vi "CTRE_PigeonIMU_Global.vi"(4 "32-bit Frame":i32, 6 "Set Boolean":bool, 7 "Write After Receive":T2={"PigeonState"=enum."NoComm", "FusedHeading"={"Heading"=0.0, "Valid?"=TRUE, "Fusing?"=TRUE}, "YPR"={"Yaw"=0.0, "Pitch"=0.0, "Roll"=0.0}, "Compass"={"Heading"=0.0, "Magnitude"=0.0, "Absolute Heading"=0.0}, "Accelerometer"={"Biased"={"X"=0, "Y"=0, "Z"=0, "Norm"=0}, "Angles"={"XZ Tilt"=0.0, "YZ Tilt"=0.0, "XY Tilt"=0.0}}, "Magnetometer"={"Raw"={"X"=0, "Y"=0, "Z"=0}, "Biased"={"X"=0, "Y"=0, "Z"=0}}, "Gyro"={"X"=0.0, "Y"=0.0, "Z"=0.0, "Norm"=0.0}, "6D Quaternian"={"W"=0.0, "X"=0.0, "Y"=0.0, "Z"=0.0}, "Temp. (C)"=0.0, "UpTime"=0, "StartupStatus"={"ResetCount"=0, "ResetFlags"=0, "FirmwareVersion"=0, "HasReset?"=TRUE}, "Calibration"={"CurrentMode"=0, "LastCalError"=0, "CalBooting?"=TRUE}, "CAN Error"={"status"=FALSE, "code"=0, "source"=""}, "AccumGyro"={"X"=0.0, "Y"=0.0, "Z"=0.0}, "Usage Frame"=0} {"Calibration"."CurrentMode" items=["BootTareGryoAccel"=0, "Temperature"=1, "Magnetometer12Pt"=2, "Magnetometer360"=3, "Accelerometer"=5]}, 8 "Set Number":dbl, 10 "Operation":T1, 11 "Device ID (0)":u8) -> (1 "Get All":T2={"PigeonState"=enum."NoComm", "FusedHeading"={"Heading"=0.0, "Valid?"=TRUE, "Fusing?"=TRUE}, "YPR"={"Yaw"=0.0, "Pitch"=0.0, "Roll"=0.0}, "Compass"={"Heading"=0.0, "Magnitude"=0.0, "Absolute Heading"=0.0}, "Accelerometer"={"Biased"={"X"=0, "Y"=0, "Z"=0, "Norm"=0}, "Angles"={"XZ Tilt"=0.0, "YZ Tilt"=0.0, "XY Tilt"=0.0}}, "Magnetometer"={"Raw"={"X"=0, "Y"=0, "Z"=0}, "Biased"={"X"=0, "Y"=0, "Z"=0}}, "Gyro"={"X"=0.0, "Y"=0.0, "Z"=0.0, "Norm"=0.0}, "6D Quaternian"={"W"=0.0, "X"=0.0, "Y"=0.0, "Z"=0.0}, "Temp. (C)"=0.0, "UpTime"=0, "StartupStatus"={"ResetCount"=0, "ResetFlags"=0, "FirmwareVersion"=0, "HasReset?"=TRUE}, "Calibration"={"CurrentMode"=0, "LastCalError"=0, "CalBooting?"=TRUE}, "CAN Error"={"status"=FALSE, "code"=0, "source"=""}, "AccumGyro"={"X"=0.0, "Y"=0.0, "Z"=0.0}, "Usage Frame"=0} {"Calibration"."CurrentMode" items=["BootTareGryoAccel"=0, "Temperature"=1, "Magnetometer12Pt"=2, "Magnetometer360"=3, "Accelerometer"=5]}, 3 "Device ID Out":u8, 5 "Read For Send":T5)   [LabVIEW 2016]
uses:
  <vilib>/Rock Robotics/WPI/ThirdParty/Sensors/Pigeon IMU/CTRE_PigeonIMU_GlobalControl.ctl
  <vilib>/Rock Robotics/WPI/ThirdParty/Sensors/Pigeon IMU/CTRE_PigeonIMU_GlobalStatus.ctl
  <vilib>/Rock Robotics/WPI/ThirdParty/Sensors/Pigeon IMU/CTRE_PigeonIMU_PigeonState.ctl
  <vilib>/Rock Robotics/WPI/ThirdParty/Sensors/Pigeon IMU/CTRE_PigeonIMU_CalibrationMode.ctl
  <vilib>/Rock Robotics/WPI/ThirdParty/Sensors/Pigeon IMU/CTRE_PigeonIMU_GlobalOps.ctl
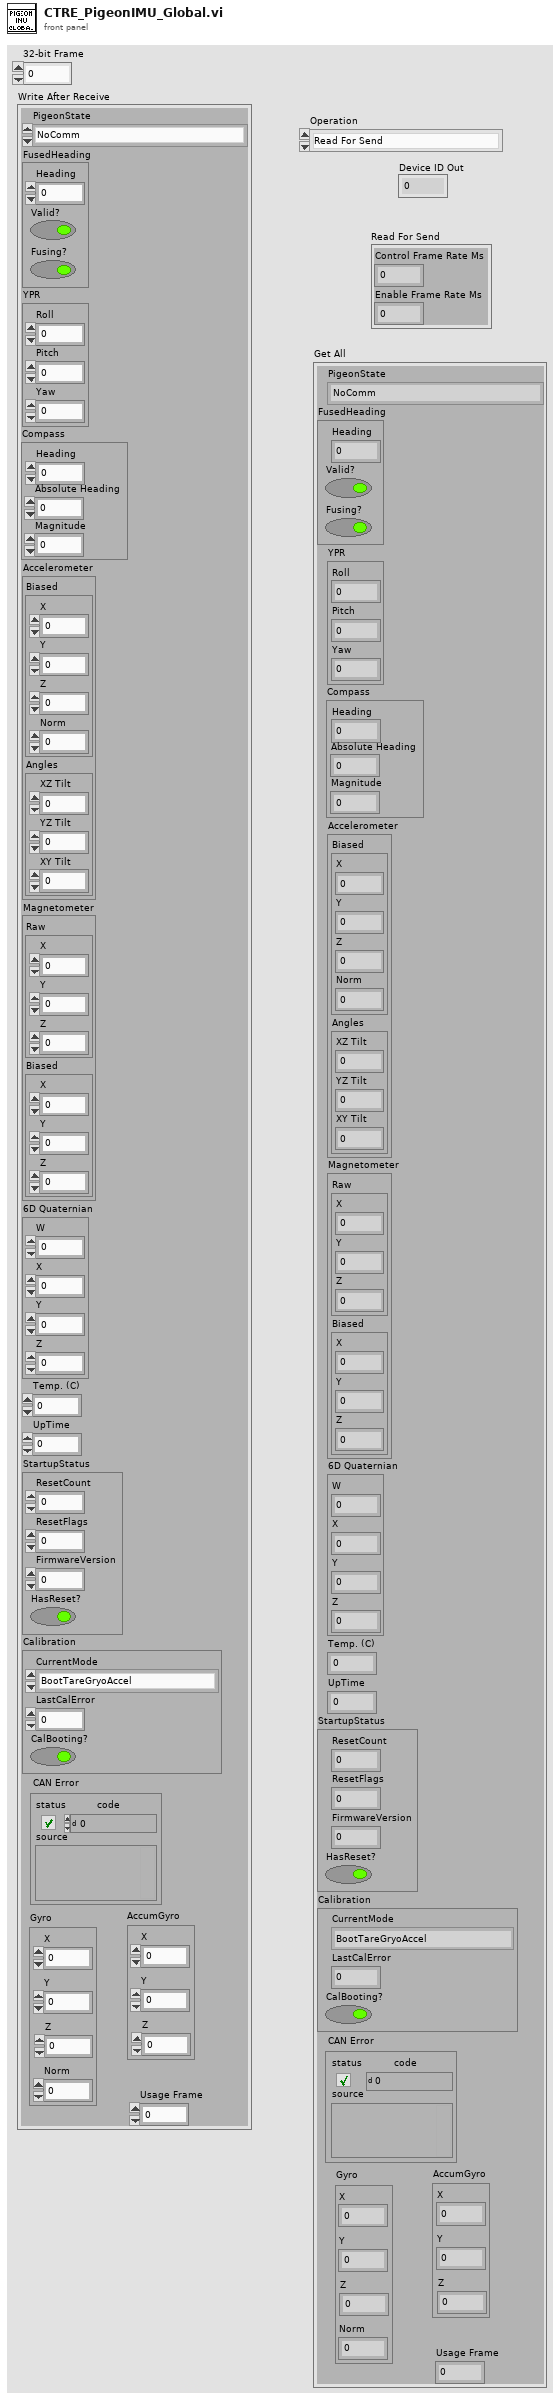
[diagram p1: front panel]
types:
  T1 = typedef "CTRE_PigeonIMU_GlobalOps.ctl" = enum16{"Read For Send", "Write Error", "Get All", "Set Control Frame Rate", "Set Enable Frame Rate", "Write After Receive Fused Heading", "Write After Receive YPR", "Write After Receive Status", "Write After Receive Raw Magnetomoter", "Write After Receive Biased Magnetometer", "Write After Receive Biased Accelerometer", "Write After Receive Gyro", "Write After Receive Acceleromter Angles", "Write After Receive Startup Status", "Write After Receive Compass", "Write After Receive Quaternian", "Write After Receive AccumGyro", "Set Usage Frame"}
  T2 = typedef "CTRE_PigeonIMU_GlobalStatus.ctl" = cluster{"PigeonState":T3, "FusedHeading":cluster{"Heading":dbl, "Valid?":bool, "Fusing?":bool}, "YPR":cluster{"Yaw":dbl, "Pitch":dbl, "Roll":dbl}, "Compass":cluster{"Heading":dbl, "Magnitude":dbl, "Absolute Heading":dbl}, "Accelerometer":cluster{"Biased":cluster{"X":i16, "Y":i16, "Z":i16, "Norm":i16}, "Angles":cluster{"XZ Tilt":dbl, "YZ Tilt":dbl, "XY Tilt":dbl}}, "Magnetometer":cluster{"Raw":cluster{"X":i16, "Y":i16, "Z":i16}, "Biased":cluster{"X":i16, "Y":i16, "Z":i16}}, "Gyro":cluster{"X":dbl, "Y":dbl, "Z":dbl, "Norm":dbl}, "6D Quaternian":cluster{"W":dbl, "X":dbl, "Y":dbl, "Z":dbl}, "Temp. (C)":dbl, "UpTime":u32, "StartupStatus":cluster{"ResetCount":i32, "ResetFlags":i32, "FirmwareVersion":i32, "HasReset?":bool}, "Calibration":cluster{"CurrentMode":T4, "LastCalError":i32, "CalBooting?":bool}, "CAN Error":errorcluster, "AccumGyro":cluster{"X":dbl, "Y":dbl, "Z":dbl}, "Usage Frame":u32}
  T3 = typedef "CTRE_PigeonIMU_PigeonState.ctl" = enum16{"NoComm", "Initializing", "Ready", "UserCalibration"}
  T4 = typedef "CTRE_PigeonIMU_CalibrationMode.ctl" = u16
  T5 = typedef "CTRE_PigeonIMU_GlobalControl.ctl" = cluster{"Control Frame Rate Ms":i32, "Enable Frame Rate Ms":i32}
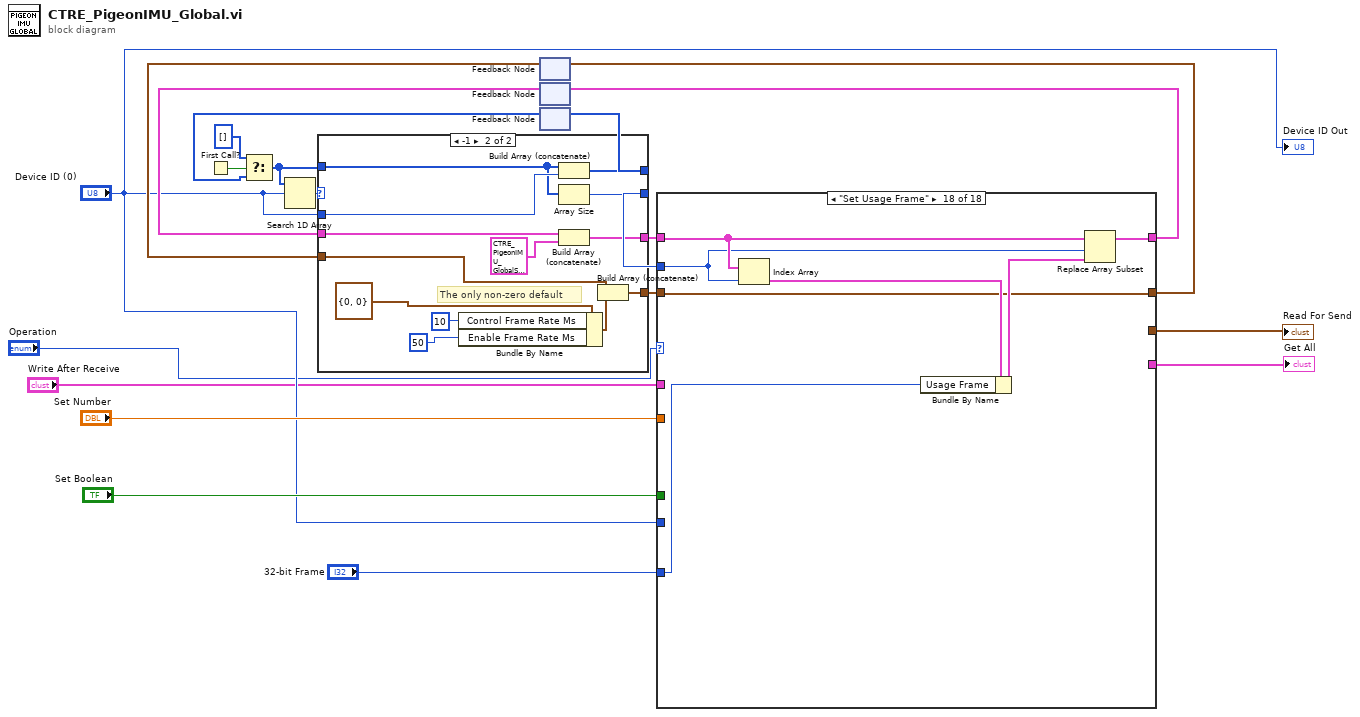
[diagram p0: block diagram]
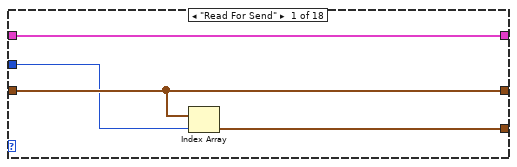
[diagram p2: hidden frame]
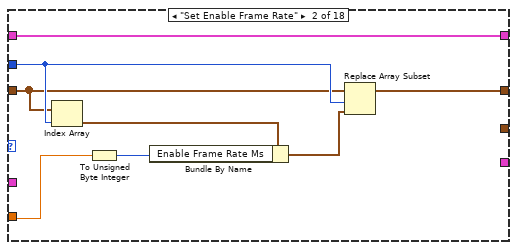
[diagram p3: hidden frame]
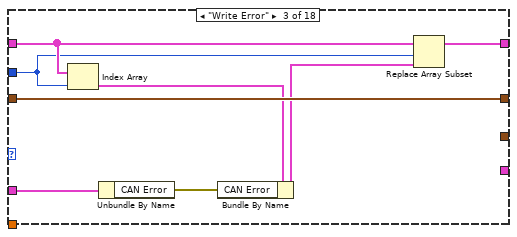
[diagram p4: hidden frame]
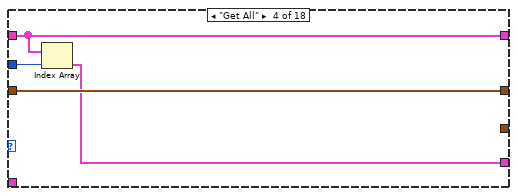
[diagram p5: hidden frame]
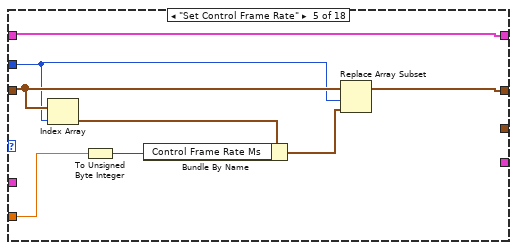
[diagram p6: hidden frame]
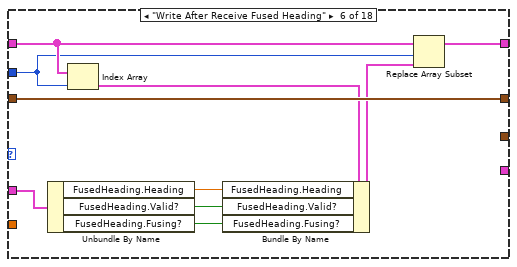
[diagram p7: hidden frame]
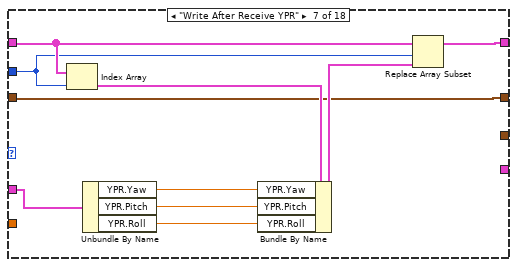
[diagram p8: hidden frame]
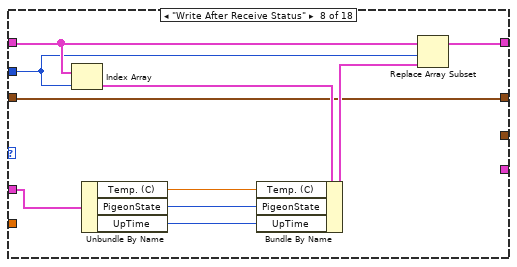
[diagram p9: hidden frame]
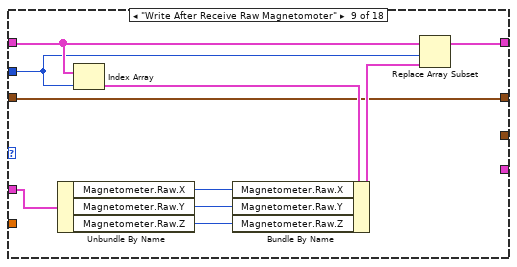
[diagram p10: hidden frame]
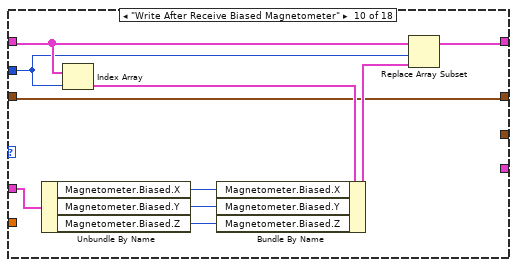
[diagram p11: hidden frame]
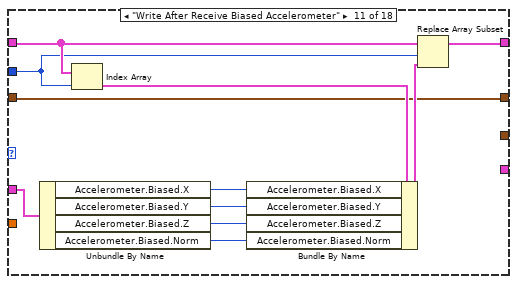
[diagram p12: hidden frame]
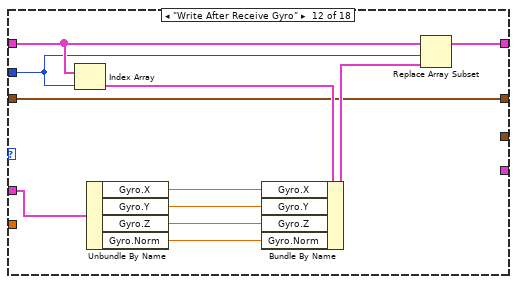
[diagram p13: hidden frame]
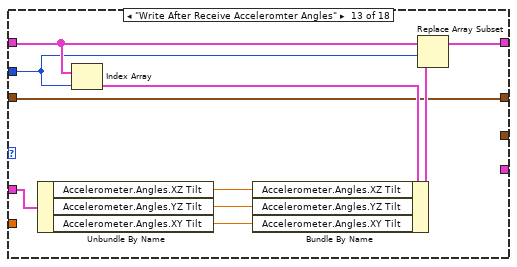
[diagram p14: hidden frame]
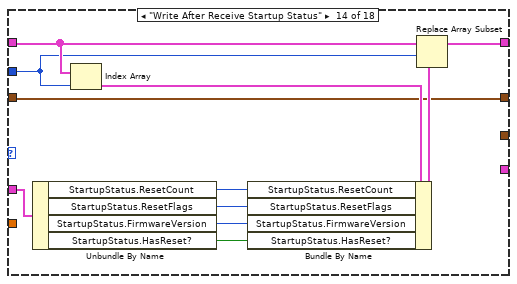
[diagram p15: hidden frame]
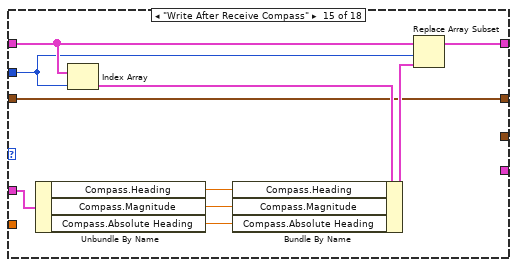
[diagram p16: hidden frame]
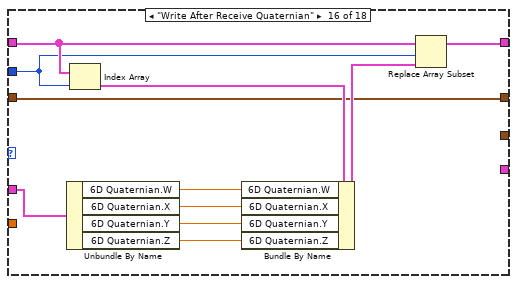
[diagram p17: hidden frame]
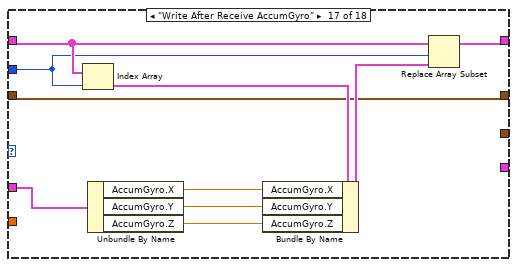
[diagram p18: hidden frame]
diagram:
  n1 = First Call?() -> (First Call?: T/F=w21:bool)
  n2 = feedback #1() -> (w14:T5[])  [unwired: 1 in]
  n3 = feedback #2() -> (w15:T2[])  [unwired: 1 in]
  n4 = feedback #3() -> (w19:u8[])  [unwired: 1 in]
  n5 = Select(t=u8[] [], s=w21, f=w19) -> (s? t:f=w17:u8[])
  n6 = Search 1D Array(1D array=w17, element="Device ID (0)") -> (index of element=w16:i32)  [unwired: 1 in]
  n7 = case shown="-1" w16 {
    selector: w16 -> [w22 _]
    tunnel: [w25 w38] -> w18
    tunnel: "Device ID (0)" -> [_ w37]
    tunnel: w17 -> [w25 w32]
    tunnel: w15 -> [w24 w36]
    tunnel: w14 -> [w23 w35]
    tunnel: [w24 w34] -> w12
    tunnel: [w23 w33] -> w10
    tunnel: [w22 w31] -> w9
    frame Default {
    }
    frame -1 {
      # "The only non-zero default"
      n8 = Bundle By Name(cluster=T5 {"Control Frame Rate Ms"=0, "Enable Frame Rate Ms"=0} ("PigeonIMU Control"), "Control Frame Rate Ms"=u8 10, "Enable Frame Rate Ms"=u8 50) -> (w30:T5)
      n9 = Build Array (concatenate)(w32, w37) -> (w38:u8[])
      n10 = Array Size(array=w32) -> (size(s)=w31:i32)
      n11 = Build Array (concatenate)(w36, T2 {"PigeonState"=enum."NoComm", "FusedHeading"={"Heading"=0.0, "Valid?"=TRUE, "Fusing?"=TRUE}, "YPR"={"Yaw"=0.0, "Pitch"=0.0, "Roll"=0.0}, "Compass"={"Heading"=0.0, "Magnitude"=0.0, "Absolute Heading"=0.0}, "Accelerometer"={"Biased"={"X"=0, "Y"=0, "Z"=0, "Norm"=0}, "Angles"={"XZ Tilt"=0.0, "YZ Tilt"=0.0, "XY Tilt"=0.0}}, "Magnetometer"={"Raw"={"X"=0, "Y"=0, "Z"=0}, "Biased"={"X"=0, "Y"=0, "Z"=0}}, "Gyro"={"X"=0.0, "Y"=0.0, "Z"=0.0, "Norm"=0.0}, "6D Quaternian"={"W"=0.0, "X"=0.0, "Y"=0.0, "Z"=0.0}, "Temp. (C)"=0.0, "UpTime"=0, "StartupStatus"={"ResetCount"=0, "ResetFlags"=0, "FirmwareVersion"=0, "HasReset?"=TRUE}, "Calibration"={"CurrentMode"=0, "LastCalError"=0, "CalBooting?"=TRUE}, "CAN Error"={"status"=FALSE, "code"=0, "source"=""}, "AccumGyro"={"X"=0.0, "Y"=0.0, "Z"=0.0}, "Usage Frame"=0} ("PigeonIMU Status")) -> (w34:T2[])
      n12 = Build Array (concatenate)(w35, w30) -> (w33:T5[])
    }
  }
  n13 = feedback-in #3(w18) -> ()
  n14 = case shown="\"Set Usage Frame\"" "Operation" {
    tunnel: [w42 w44 w57 w60 w66 w79 w84 w94 w104 w114 w125 w136 w146 w157 w168 w179 w188 w197] -> w13
    tunnel: w12 -> [w42 w44 w56 w60 w66 w78 w85 w95 w105 w115 w126 w137 w147 w158 w170 w181 w189 w199]
    tunnel: [w41 w43 w58 w62 w68 w80 w83 w92 w102 w112 w123 w134 w145 w155 w167 w178 w186 w196] -> w11
    tunnel: w10 -> [w41 w45 w58 w62 w69 w80 w83 w92 w102 w112 w123 w134 w145 w155 w167 w178 w186 w196]
    tunnel: w9 -> [w40 w46 w55 w61 w67 w77 w82 w93 w103 w113 w124 w135 w143 w156 w169 w180 w187 w198]
    tunnel: [w39 _ _ _ _ _ _ _ _ _ _ _ _ _ _ _ _ _] -> w5
    tunnel: "Write After Receive" -> [_ _ w52 _ _ w74 w81 w91 w101 w111 w122 w133 w144 w154 w166 w177 w185 _]
    tunnel: "Set Number" -> [_ w47 _ _ w64 _ _ _ _ _ _ _ _ _ _ _ _ _]
    tunnel: [_ _ _ w59 _ _ _ _ _ _ _ _ _ _ _ _ _ _] -> w4
    tunnel: "Set Boolean" -> [_ _ _ _ _ _ _ _ _ _ _ _ _ _ _ _ _ _]
    tunnel: "Device ID (0)" -> [_ _ _ _ _ _ _ _ _ _ _ _ _ _ _ _ _ _]
    tunnel: "32-bit Frame" -> [_ _ _ _ _ _ _ _ _ _ _ _ _ _ _ _ _ w195]
    frame "Read For Send" {
      n15 = Index Array(array=w41, index=w40) -> (element=w39:T5)
    }
    frame "Set Enable Frame Rate" {
      n16 = Index Array(array=w45, index=w46) -> (element=w49:T5)
      n17 = To Unsigned Byte Integer(number=w47) -> (unsigned 8bit integer=w48:u8)
      n18 = Bundle By Name(cluster=w49, "Enable Frame Rate Ms"=w48) -> (w50:T5)
      n19 = Replace Array Subset(array=w45, new element=w50, index=w46) -> (w43:T5[])
    }
    frame "Write Error" {
      n20 = Index Array(array=w56, index=w55) -> (element=w54:T2)
      n21 = Unbundle By Name(w52) -> ("CAN Error"=w51:errorcluster)
      n22 = Bundle By Name(cluster=w54, "CAN Error"=w51) -> (w53:T2)
      n23 = Replace Array Subset(array=w56, new element=w53, index=w55) -> (w57:T2[])
    }
    frame "Get All" {
      n24 = Index Array(array=w60, index=w61) -> (element=w59:T2)
    }
    frame "Set Control Frame Rate" {
      n25 = Index Array(array=w69, index=w67) -> (element=w65:T5)
      n26 = To Unsigned Byte Integer(number=w64) -> (unsigned 8bit integer=w63:u8)
      n27 = Bundle By Name(cluster=w65, "Control Frame Rate Ms"=w63) -> (w70:T5)
      n28 = Replace Array Subset(array=w69, new element=w70, index=w67) -> (w68:T5[])
    }
    frame "Write After Receive Fused Heading" {
      n29 = Unbundle By Name(w74) -> ("FusedHeading.Heading"=w73:dbl, "FusedHeading.Valid?"=w72:bool, "FusedHeading.Fusing?"=w71:bool)
      n30 = Index Array(array=w78, index=w77) -> (element=w76:T2)
      n31 = Bundle By Name(cluster=w76, "FusedHeading.Heading"=w73, "FusedHeading.Valid?"=w72, "FusedHeading.Fusing?"=w71) -> (w75:T2)
      n32 = Replace Array Subset(array=w78, new element=w75, index=w77) -> (w79:T2[])
    }
    frame "Write After Receive YPR" {
      n33 = Index Array(array=w85, index=w82) -> (element=w86:T2)
      n34 = Unbundle By Name(w81) -> ("YPR.Yaw"=w88:dbl, "YPR.Pitch"=w89:dbl, "YPR.Roll"=w90:dbl)
      n35 = Bundle By Name(cluster=w86, "YPR.Yaw"=w88, "YPR.Pitch"=w89, "YPR.Roll"=w90) -> (w87:T2)
      n36 = Replace Array Subset(array=w85, new element=w87, index=w82) -> (w84:T2[])
    }
    frame "Write After Receive Status" {
      n37 = Index Array(array=w95, index=w93) -> (element=w100:T2)
      n38 = Unbundle By Name(w91) -> ("Temp. (C)"=w98:dbl, "PigeonState"=w97:T3, "UpTime"=w96:u32)
      n39 = Bundle By Name(cluster=w100, "Temp. (C)"=w98, "PigeonState"=w97, "UpTime"=w96) -> (w99:T2)
      n40 = Replace Array Subset(array=w95, new element=w99, index=w93) -> (w94:T2[])
    }
    frame "Write After Receive Raw Magnetomoter" {
      n41 = Unbundle By Name(w101) -> ("Magnetometer.Raw.X"=w108:i16, "Magnetometer.Raw.Y"=w107:i16, "Magnetometer.Raw.Z"=w106:i16)
      n42 = Index Array(array=w105, index=w103) -> (element=w110:T2)
      n43 = Bundle By Name(cluster=w110, "Magnetometer.Raw.X"=w108, "Magnetometer.Raw.Y"=w107, "Magnetometer.Raw.Z"=w106) -> (w109:T2)
      n44 = Replace Array Subset(array=w105, new element=w109, index=w103) -> (w104:T2[])
    }
    frame "Write After Receive Biased Magnetometer" {
      n45 = Unbundle By Name(w111) -> ("Magnetometer.Biased.X"=w118:i16, "Magnetometer.Biased.Y"=w117:i16, "Magnetometer.Biased.Z"=w116:i16)
      n46 = Index Array(array=w115, index=w113) -> (element=w120:T2)
      n47 = Bundle By Name(cluster=w120, "Magnetometer.Biased.X"=w118, "Magnetometer.Biased.Y"=w117, "Magnetometer.Biased.Z"=w116) -> (w119:T2)
      n48 = Replace Array Subset(array=w115, new element=w119, index=w113) -> (w114:T2[])
    }
    frame "Write After Receive Biased Accelerometer" {
      n49 = Unbundle By Name(w122) -> ("Accelerometer.Biased.X"=w129:i16, "Accelerometer.Biased.Y"=w128:i16, "Accelerometer.Biased.Z"=w127:i16, "Accelerometer.Biased.Norm"=w121:i16)
      n50 = Index Array(array=w126, index=w124) -> (element=w131:T2)
      n51 = Bundle By Name(cluster=w131, "Accelerometer.Biased.X"=w129, "Accelerometer.Biased.Y"=w128, "Accelerometer.Biased.Z"=w127, "Accelerometer.Biased.Norm"=w121) -> (w130:T2)
      n52 = Replace Array Subset(array=w126, new element=w130, index=w124) -> (w125:T2[])
    }
    frame "Write After Receive Gyro" {
      n53 = Index Array(array=w137, index=w135) -> (element=w142:T2)
      n54 = Unbundle By Name(w133) -> ("Gyro.X"=w140:dbl, "Gyro.Y"=w139:dbl, "Gyro.Z"=w138:dbl, "Gyro.Norm"=w132:dbl)
      n55 = Bundle By Name(cluster=w142, "Gyro.X"=w140, "Gyro.Y"=w139, "Gyro.Z"=w138, "Gyro.Norm"=w132) -> (w141:T2)
      n56 = Replace Array Subset(array=w137, new element=w141, index=w135) -> (w136:T2[])
    }
    frame "Write After Receive Acceleromter Angles" {
      n57 = Unbundle By Name(w144) -> ("Accelerometer.Angles.XZ Tilt"=w150:dbl, "Accelerometer.Angles.YZ Tilt"=w151:dbl, "Accelerometer.Angles.XY Tilt"=w152:dbl)
      n58 = Index Array(array=w147, index=w143) -> (element=w148:T2)
      n59 = Bundle By Name(cluster=w148, "Accelerometer.Angles.XZ Tilt"=w150, "Accelerometer.Angles.YZ Tilt"=w151, "Accelerometer.Angles.XY Tilt"=w152) -> (w149:T2)
      n60 = Replace Array Subset(array=w147, new element=w149, index=w143) -> (w146:T2[])
    }
    frame "Write After Receive Startup Status" {
      n61 = Unbundle By Name(w154) -> ("StartupStatus.ResetCount"=w161:i32, "StartupStatus.ResetFlags"=w160:i32, "StartupStatus.FirmwareVersion"=w159:i32, "StartupStatus.HasReset?"=w153:bool)
      n62 = Index Array(array=w158, index=w156) -> (element=w163:T2)
      n63 = Bundle By Name(cluster=w163, "StartupStatus.ResetCount"=w161, "StartupStatus.ResetFlags"=w160, "StartupStatus.FirmwareVersion"=w159, "StartupStatus.HasReset?"=w153) -> (w162:T2)
      n64 = Replace Array Subset(array=w158, new element=w162, index=w156) -> (w157:T2[])
    }
    frame "Write After Receive Compass" {
      n65 = Unbundle By Name(w166) -> ("Compass.Heading"=w173:dbl, "Compass.Magnitude"=w165:dbl, "Compass.Absolute Heading"=w164:dbl)
      n66 = Index Array(array=w170, index=w169) -> (element=w171:T2)
      n67 = Bundle By Name(cluster=w171, "Compass.Heading"=w173, "Compass.Magnitude"=w165, "Compass.Absolute Heading"=w164) -> (w172:T2)
      n68 = Replace Array Subset(array=w170, new element=w172, index=w169) -> (w168:T2[])
    }
    frame "Write After Receive Quaternian" {
      n69 = Unbundle By Name(w177) -> ("6D Quaternian.W"=w182:dbl, "6D Quaternian.X"=w176:dbl, "6D Quaternian.Y"=w175:dbl, "6D Quaternian.Z"=w174:dbl)
      n70 = Index Array(array=w181, index=w180) -> (element=w184:T2)
      n71 = Bundle By Name(cluster=w184, "6D Quaternian.W"=w182, "6D Quaternian.X"=w176, "6D Quaternian.Y"=w175, "6D Quaternian.Z"=w174) -> (w183:T2)
      n72 = Replace Array Subset(array=w181, new element=w183, index=w180) -> (w179:T2[])
    }
    frame "Write After Receive AccumGyro" {
      n73 = Index Array(array=w189, index=w187) -> (element=w190:T2)
      n74 = Unbundle By Name(w185) -> ("AccumGyro.X"=w192:dbl, "AccumGyro.Y"=w193:dbl, "AccumGyro.Z"=w194:dbl)
      n75 = Bundle By Name(cluster=w190, "AccumGyro.X"=w192, "AccumGyro.Y"=w193, "AccumGyro.Z"=w194) -> (w191:T2)
      n76 = Replace Array Subset(array=w189, new element=w191, index=w187) -> (w188:T2[])
    }
    frame "Set Usage Frame" {
      n77 = Index Array(array=w199, index=w198) -> (element=w200:T2)
      n78 = Bundle By Name(cluster=w200, "Usage Frame"=w195) -> (w201:T2)
      n79 = Replace Array Subset(array=w199, new element=w201, index=w198) -> (w197:T2[])
    }
  }
  "Read For Send" <- w5
  "Get All" <- w4
  n80 = feedback-in #1(w11) -> ()
  n81 = feedback-in #2(w13) -> ()
  "Device ID Out" <- "Device ID (0)"
